vi "getMotRng.vi"(8 "error in (no error)":errorcluster, 10 "Rigid Body Stroke File":string="rbStroke.txt", 11 "OptCtrl in":refnum<class "OptCtrl.lvclass">) -> (0 "error out":errorcluster, 2 "Range of DOF":dbl[](array[numeric]), 3 "OptCtrl out":refnum<class "OptCtrl.lvclass">)   [LabVIEW 2016, in "OptCtrl.lvclass"]
doc: "Get the range of motion of degree of freedom (DOF)."
uses:
  OptCtrl.lvclass
  OptCtrl.lvclass/OptCtrl.ctl
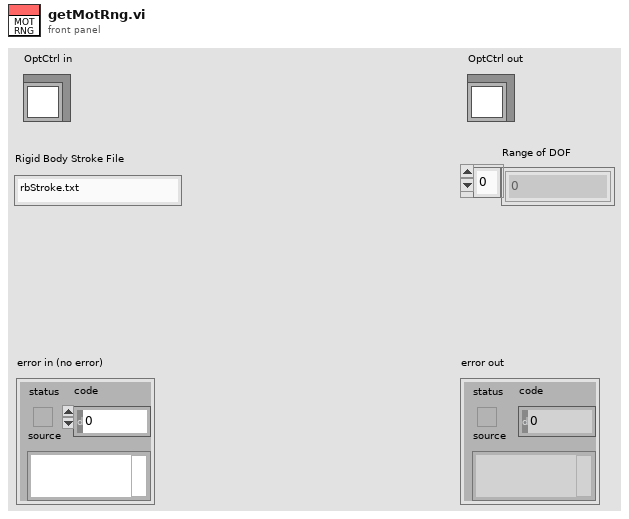
[diagram p1: front panel]
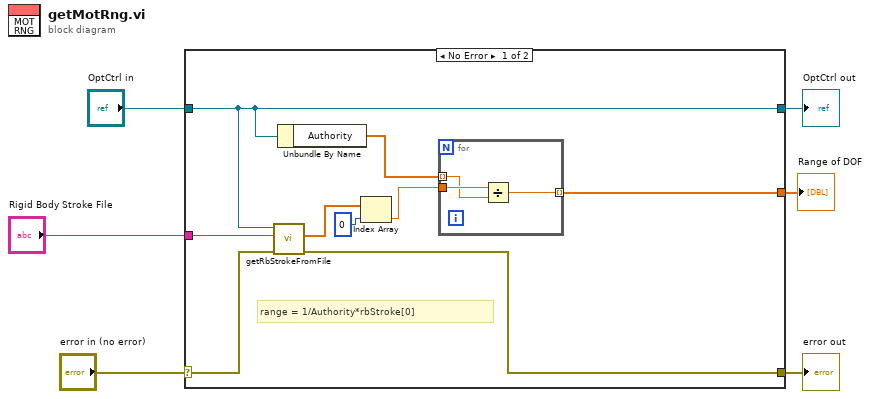
[diagram p0: block diagram]
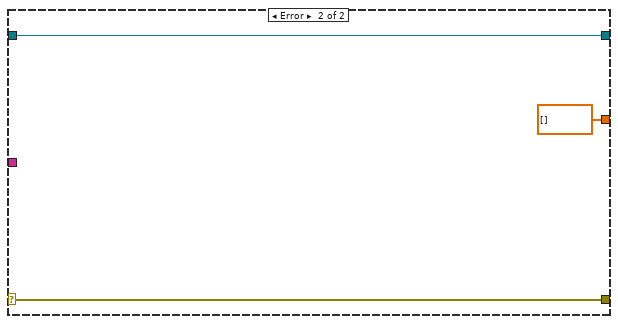
[diagram p2: hidden frame]
diagram:
  n1 = case shown="No Error" "error in (no error)" {
    selector: "error in (no error)" -> [w13 w21]
    tunnel: [w12 w21] -> w5
    tunnel: [w15 w20] -> w4
    tunnel: "OptCtrl in" -> [w15 w20]
    tunnel: "Rigid Body Stroke File" -> [w14 _]
    tunnel: [w7 dbl[] []] -> w2
    frame No Error {
      # "range = 1/Authority*rbStroke[0]"
      n2 = call "getRbStrokeFromFile.vi"("error in (no error)"=w13, "Rigid Body Stroke File"=w14, "OptCtrl in"=w15) -> ("error out"=w12:errorcluster, "Stroke in Um"=w11:dbl[])  [unwired: 6 in, 1 out]
      n3 = Unbundle By Name(w15) -> ("Authority"=w9:dbl[])
      n4 = Index Array(array=w11, index=0) -> (element=w8:dbl)
      n5 = for {
        tunnel: w9 -> [w17] mode=indexing
        tunnel: w8 -> [w18]
        tunnel: [w16] -> w7 mode=indexing
        n6 = Divide(x=w18, y=w17) -> (x/y=w16:dbl)
      }
    }
    frame Error {
    }
  }
  "error out" <- w5
  "OptCtrl out" <- w4
  "Range of DOF" <- w2
